vi "Memory.Pointer.Read Bytes.Subset.vi"   [LabVIEW 2016, in "Memory Manager.lvlib" / "Memory.Pointer.Void.lvclass"]
uses:
  Memory.Pointer.Void.lvclass
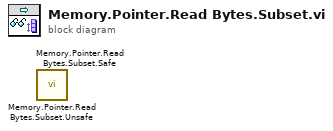
[diagram p0: block diagram]
diagram:
  n1 = call "Memory.Pointer.Read Bytes.Subset.Unsafe.vi"() -> ()  [unwired: 8 in, 4 out]
  n2 = call "Memory.Pointer.Read Bytes.Subset.Safe.vi"() -> ()  [unwired: 8 in, 4 out]
